vi "SubVI_ProcessTitle.vi"(11 "Title":string[](array[string])) -> (3 "Array":T1[](array[typedef]))   [LabVIEW 2012]
uses:
  Data File Processing UI_ChannelSet.ctl
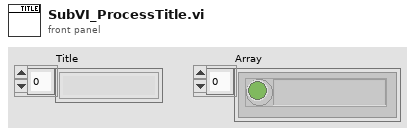
[diagram p1: front panel]
types:
  T1 = typedef "Data File Processing UI_ChannelSet.ctl" = cluster{"Select":bool, "Channel":string}
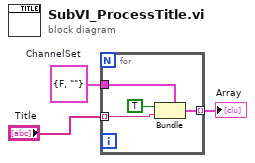
[diagram p0: block diagram]
diagram:
  w2 = T1 {"Select"=FALSE, "Channel"=""}  # ChannelSet
  n1 = for {
    tunnel: "Title" -> [w6] mode=indexing
    tunnel: w2 -> [w5]
    tunnel: [w4] -> w3 mode=indexing
    n2 = Bundle(cluster=w5, "Select"=TRUE, "Channel"=w6) -> (w4:T1)
  }
  "Array" <- w3
